vi "Magspec cam1 ana_for_Hann.vi"(3 "Image I16":i16[][](array[numeric])=array512x384[196608 elements], 4 "confg cluster":T1={"position"=45.72, "field of view"=106.18, "Analysis ROI"=[0, 0, 512, 384]}, 5 "true4Fwd":bool=TRUE, 6 "B [mT]":dbl=816.6739225545333 format="%#_3g") -> (0 "XY Graph":cluster{"energy":dbl[], "counts":dbl[]}(graph), 1 "Peak location":dbl=166.5382748228936, 2 "dE/E":dbl=0.6853812640250416)   [LabVIEW 2013]
panel:
  in  "input cluster":cluster{"energy":dbl[], "counts":dbl[]}
  out "sum":i64=-4664
  out "MSData0":dbl[](array[numeric])=[40.10396835354356, nan, 75.2707975986278, 45.106732064958535, -4664.0]
  out "min value":dbl=88.25253291892105
  out "max value":dbl=226.00939455537824
  out "saveXpixel":i32=512
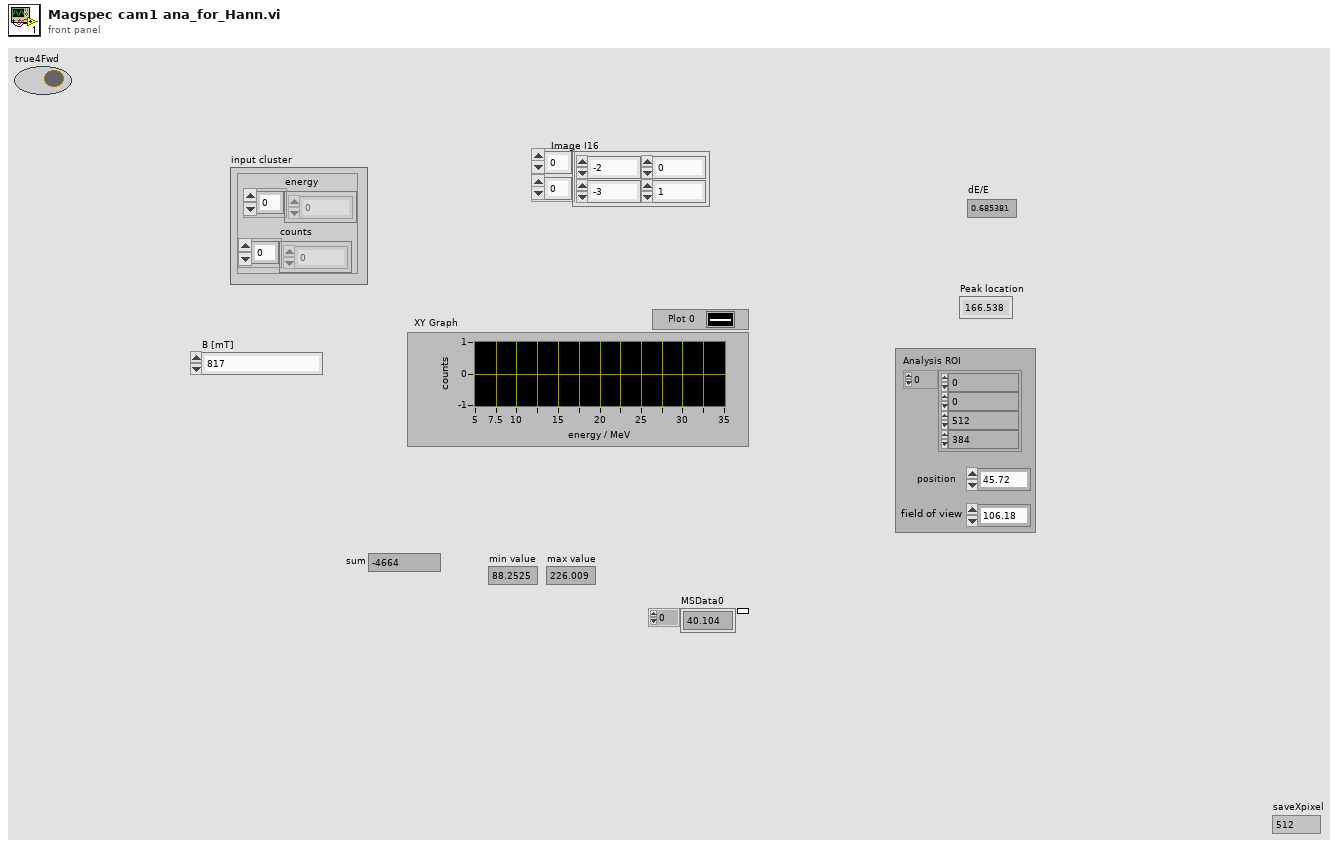
[diagram p1: front panel]
types:
  T1 = cluster{"position":dbl, "field of view":dbl, "Analysis ROI":i32[]}
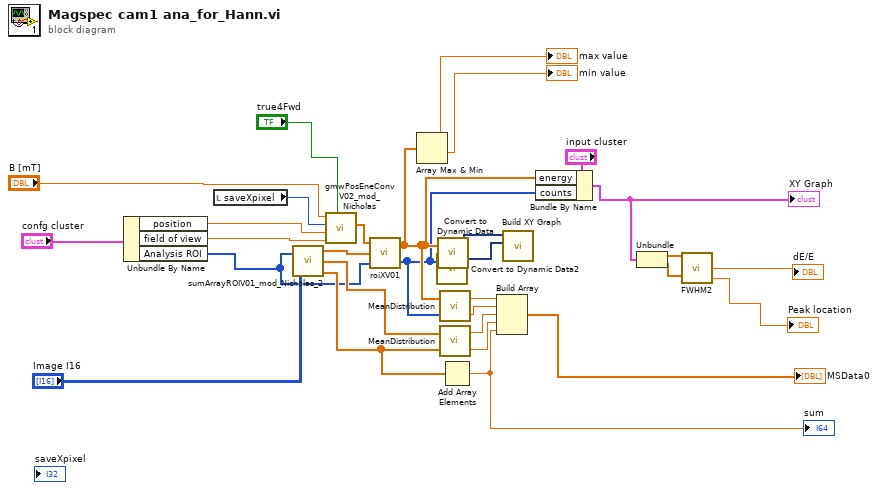
[diagram p0: block diagram]
diagram:
  n1 = Unbundle By Name("confg cluster") -> ("position"=w24:dbl, "field of view"=w25:dbl, "Analysis ROI"=w2:i32[])
  n2 = local read "saveXpixel"() -> (w26:i32)
  n3 = call "sumArrayROIV01_mod_Nicholas_2.vi"("ROI"=w2, "Image I16"="Image I16") -> ("EDist"=w27:dbl[], "Aaxis"=w19:dbl[], "ADist"=w14:dbl[])
  n4 = call "gmwPosEneConvV02_mod_Nicholas.vi"("true4Fwd"="true4Fwd", "field of view"=w25, "position"=w24, "pixel number"=w26, "b[mT]"="B [mT]") -> ("energy [MeV]"=w28:dbl[])  [unwired: 4 out]
  n5 = call "roiXV01.vi"("ROI"=w2, "ArrayY"=w27, "ArrayX"=w28) -> ("yOut"=w6:i32[], "xOut"=w7:dbl[])
  n6 = Array Max & Min(array=w7) -> (max value=→"max value":dbl, min value=→"min value":dbl)  [unwired: 2 out]
  n7 = call "Convert to Dynamic Data2"("Array"=w6) -> ("Dynamic Data Type"=w29:dynamicdata)  [unwired: 3 out]
  n8 = call "Convert to Dynamic Data"("Array"=w7) -> ("Dynamic Data Type"=w30:dynamicdata)  [unwired: 3 out]
  n9 = call "MeanDistribution.vi"("y=f(x)"=w6, "x"=w7) -> ("Std of Distribution"=w20:dbl, "Mean of distribution"=w21:dbl)
  n10 = call "MeanDistribution.vi"("y=f(x)"=w14, "x"=w19) -> ("Std of Distribution"=w17:dbl, "Mean of distribution"=w18:dbl)
  n11 = Add Array Elements(numeric array=w14) -> (sum=w15:dbl)
  "sum" <- w15
  n12 = Build Array(w21, w20, w18, w17, w15) -> (→"MSData0":dbl[])
  n13 = call "Build XY Graph"("Y Input"=w29, "X Input"=w30) -> ()  [unwired: 3 in, 7 out]
  n14 = Bundle By Name(cluster="input cluster", "energy"=w7, "counts"=w6) -> (w4:cluster{"energy":dbl[], "counts":dbl[]})
  "XY Graph" <- w4
  n15 = Unbundle(w4) -> ("energy"=w11:dbl[], "counts"=w10:dbl[])
  n16 = call "FWHM2.vi"("Input X"=w11, "Inpput Y"=w10) -> ("dE/E"=→"dE/E":dbl, "X Peak location"=→"Peak location":dbl)  [unwired: 1 out]
